vi "Bundle SV.vi"(8 "error in (no error)":errorcluster, 10 "Process Name":string="Flow Module 1", 11 "State Cluster in":T1={"Settings"={"Hardware Configuration"={"Tasks Array"=[]}, "Logging Configuration"={"Log File Base Path"=path ""}, "Feed Module Configuration"={"Cycle Period"=0.0, "Ismatech"={"VISA resource name"="", "Simulated?"=FALSE, "Pump Number"=0.0, "Reverse?"=FALSE}, "Masterflex"={"VISA resource name"="", "Simulated?"=FALSE, "Pump Number"=1.0, "Reverse?"=FALSE}, "Mettler"={"VISA resource name"="", "Simulated?"=FALSE}, "Bronkhorst M13 Flow Meter"={"VISA resource name"="", "Simulated?"=FALSE, "Smoothing Steps"=1}, "PID 2 Parameters"={"Input Device"=enum."Flowmeter", "Output Device"=enum."Ismatec ISM 831C", "Setpoint"=0.0, "PID gains"={"proportional gain (Kc)"=1.0, "integral time (Ti, min)"=0.01, "derivative time (Td, min)"=0.0}}, "Manual Entry"=0.0, "Auto?"=TRUE, "VICI Settings"={"VISA resource name"="", "Simulated?"=FALSE, "Pump Number"=0.0, "Reverse?"=FALSE}, "output range"={"output high"=100.0, "output low"=0.0}}, "Load Count"=0.0, "TT Configuration In"={"physical channels"="cDAQ2Mod4/ai0", "name to assign"="", "units"=10143}, "PT Configuration"={"physical channels"="cDAQ2Mod8/ai15", "name to assign"="Pressure", "units"=10342}}, "Shared Variables"={"PID 1 Process Variable"="PID1-Mettler Toledo Scale 1", "PID 1 Output"="PID1-Mettler Toledo Scale 1", "PID 1 Setpoint"="PID1-Setpoint", "PID 1 Setpoint SV refnum"="ni.var.psp://localhost/Flow Module 1/PID1-Setpoint", "PID 1 Process Variable SV refnum"="ni.var.psp://localhost/Flow Module 1/PID1-Setpoint", "PID 1 Output SV refnum"="ni.var.psp://localhost/Flow Module 1/PID1-Setpoint"}} {"Settings"."PT Configuration"."units" items=["Amps"=10342, "From Custom Scale"=10065]; "Settings"."TT Configuration In"."units" items=["Deg C"=10143, "Deg F"=10144, "Kelvins"=10325, "Deg R"=10145, "From Custom Scale"=10065]; "Settings"."Feed Module Configuration"."output range"."output low" min=0.0 max=100.0 format="%.2f"; "Settings"."Feed Module Configuration"."output range"."output high" format="%.2f"; "Settings"."Feed Module Configuration"."VICI Settings"."Pump Number" min=1.0 max=20.0 step=1.0; "Settings"."Feed Module Configuration"."PID 2 Parameters"."PID gains"."derivative time (Td, min)" format="%.3f"; "Settings"."Feed Module Configuration"."PID 2 Parameters"."PID gains"."integral time (Ti, min)" format="%.3f"; "Settings"."Feed Module Configuration"."PID 2 Parameters"."PID gains"."proportional gain (Kc)" format="%.3f"; "Settings"."Feed Module Configuration"."Bronkhorst M13 Flow Meter"."Smoothing Steps" min=1 step=1; "Settings"."Feed Module Configuration"."Masterflex"."Pump Number" min=1.0 max=20.0 step=1.0; "Settings"."Feed Module Configuration"."Ismatech"."Pump Number" min=1.0 max=20.0 step=1.0}) -> (0 "error out":errorcluster, 3 "State Cluster out":T1={"Settings"={"Hardware Configuration"={"Tasks Array"=[]}, "Logging Configuration"={"Log File Base Path"=path ""}, "Feed Module Configuration"={"Cycle Period"=0.0, "Ismatech"={"VISA resource name"="", "Simulated?"=FALSE, "Pump Number"=0.0, "Reverse?"=FALSE}, "Masterflex"={"VISA resource name"="", "Simulated?"=FALSE, "Pump Number"=1.0, "Reverse?"=FALSE}, "Mettler"={"VISA resource name"="", "Simulated?"=FALSE}, "Bronkhorst M13 Flow Meter"={"VISA resource name"="", "Simulated?"=FALSE, "Smoothing Steps"=1}, "PID 2 Parameters"={"Input Device"=enum."Flowmeter", "Output Device"=enum."Ismatec ISM 831C", "Setpoint"=0.0, "PID gains"={"proportional gain (Kc)"=1.0, "integral time (Ti, min)"=0.01, "derivative time (Td, min)"=0.0}}, "Manual Entry"=0.0, "Auto?"=TRUE, "VICI Settings"={"VISA resource name"="", "Simulated?"=FALSE, "Pump Number"=0.0, "Reverse?"=FALSE}, "output range"={"output high"=100.0, "output low"=0.0}}, "Load Count"=0.0, "TT Configuration In"={"physical channels"="cDAQ2Mod4/ai0", "name to assign"="", "units"=10143}, "PT Configuration"={"physical channels"="cDAQ2Mod8/ai15", "name to assign"="Pressure", "units"=10342}}, "Shared Variables"={"PID 1 Process Variable"="PID1-Mettler Toledo Scale 1", "PID 1 Output"="PID1-Mettler Toledo Scale 1", "PID 1 Setpoint"="PID1-Setpoint", "PID 1 Setpoint SV refnum"="ni.var.psp://localhost/Flow Module 1/PID1-Setpoint", "PID 1 Process Variable SV refnum"="ni.var.psp://localhost/Flow Module 1/PID1-Setpoint", "PID 1 Output SV refnum"="ni.var.psp://localhost/Flow Module 1/PID1-Setpoint"}} {"Settings"."PT Configuration"."units" items=["Amps"=10342, "From Custom Scale"=10065]; "Settings"."TT Configuration In"."units" items=["Deg C"=10143, "Deg F"=10144, "Kelvins"=10325, "Deg R"=10145, "From Custom Scale"=10065]; "Settings"."Feed Module Configuration"."output range"."output low" min=0.0 max=100.0 format="%.2f"; "Settings"."Feed Module Configuration"."output range"."output high" format="%.2f"; "Settings"."Feed Module Configuration"."VICI Settings"."Pump Number" min=1.0 max=20.0 step=1.0; "Settings"."Feed Module Configuration"."PID 2 Parameters"."PID gains"."derivative time (Td, min)" format="%.3f"; "Settings"."Feed Module Configuration"."PID 2 Parameters"."PID gains"."integral time (Ti, min)" format="%.3f"; "Settings"."Feed Module Configuration"."PID 2 Parameters"."PID gains"."proportional gain (Kc)" format="%.3f"; "Settings"."Feed Module Configuration"."Bronkhorst M13 Flow Meter"."Smoothing Steps" min=1 step=1; "Settings"."Feed Module Configuration"."Masterflex"."Pump Number" min=1.0 max=20.0 step=1.0; "Settings"."Feed Module Configuration"."Ismatech"."Pump Number" min=1.0 max=20.0 step=1.0})   [LabVIEW 2021, in "Scale Module.lvlib"]
uses:
  Scale Module.lvlib
  Shared Variables/Dynamic Shared Variables.lvlib
  Controls/Scale Module Shared Variable Cluster.ctl
  Acquisition/Hardware Configuration.ctl
  DAQ/DAQ.lvlib
  Logging/Logging Configuration.ctl
  Logging/Logging.lvlib
  Controls/Scale Module Settings Cluster.ctl
  Settings/Settings.ctl
  Settings/Settings.lvlib
  Controls/Scale Module State Cluster.ctl
  Masterflex 7550-30/Controls/Settings Cluster.ctl
  Masterflex 7550-30/Masterflex 7550-30.lvlib
  Mettler Toledo/Controls/Settings Cluster.ctl
  Mettler Toledo/Mettler Toledo.lvlib
  Bronkhorst M13 Flow Meter/Settings Cluster.ctl
  Bronkhorst M13 Flow Meter/Bronkhorst M13 Flow Meter.lvlib
  Measure Instrument/PID Input Enum.ctl
  Measure Instrument/PID 2 Output Enum.ctl
  Measure Instrument/PID 2 Parameters Cluster.ctl
  Ismatec ISM 831C/Controls/Ismatech Settings Cluster.ctl
  Pressure Sensor/PT Configuration.ctl
  Pressure Sensor/Pressure.lvlib
  Acquisition/Task Cluster.ctl
  VICI M50/VICI Settings.ctl
panel:
  # "Output Instruments"
  # "Input Instruments"
  # "Output Instruments"
  # "Input Instruments"
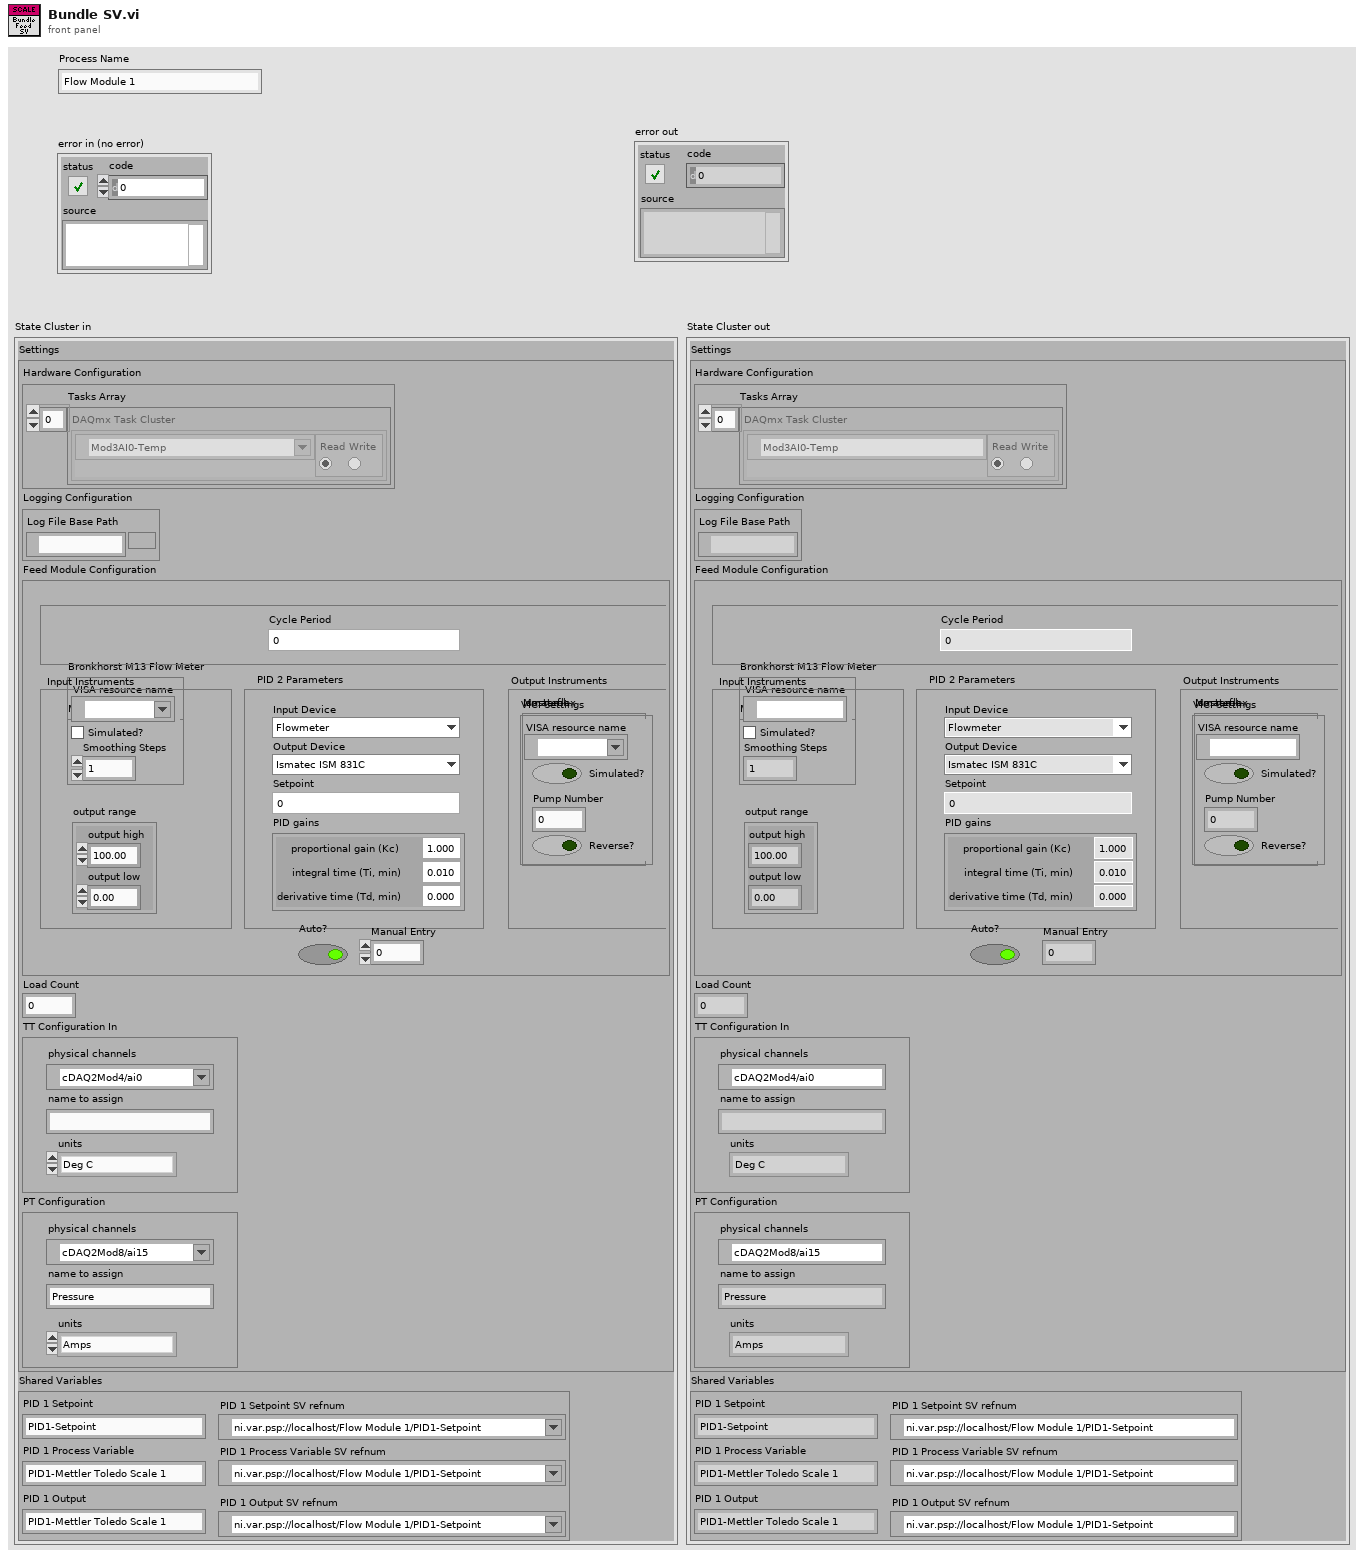
[diagram p1: front panel]
types:
  T1 = typedef "Scale Module.lvlib/Scale Module State Cluster.ctl" = cluster{"Settings":T2, "Shared Variables":T16}
  T2 = typedef "Settings.lvlib/Settings.ctl" = cluster{"Hardware Configuration":T3, "Logging Configuration":T5, "Feed Module Configuration":T6, "Load Count":dbl, "TT Configuration In":cluster{"physical channels":tag, "name to assign":string, "units":i32}, "PT Configuration":T15}
  T3 = typedef "DAQ.lvlib/Hardware Configuration.ctl" = cluster{"Tasks Array":T4[]}
  T4 = typedef "Task Cluster.ctl" = cluster{"DAQmx Task":refnum<k21>, "Read-Write Radio":enum32{"Read", "Write"}}
  T5 = typedef "Logging.lvlib/Logging Configuration.ctl" = cluster{"Log File Base Path":path}
  T6 = typedef "Scale Module.lvlib/Scale Module Settings Cluster.ctl" = cluster{"Cycle Period":dbl, "Ismatech":T7, "Masterflex":T8, "Mettler":T9, "Bronkhorst M13 Flow Meter":T10, "PID 2 Parameters":T11, "Manual Entry":dbl, "Auto?":bool, "VICI Settings":T14, "output range":cluster{"output high":dbl, "output low":dbl}}
  T7 = typedef "Ismatec ISM 831C.lvlib/Ismatech Settings Cluster.ctl" = cluster{"VISA resource name":refnum<visa-resource-name>, "Simulated?":bool, "Pump Number":dbl, "Reverse?":bool}
  T8 = typedef "Masterflex 7550-30.lvlib/Settings Cluster.ctl" = cluster{"VISA resource name":refnum<visa-resource-name>, "Simulated?":bool, "Pump Number":dbl, "Reverse?":bool}
  T9 = typedef "Mettler Toledo.lvlib/Settings Cluster.ctl" = cluster{"VISA resource name":refnum<visa-resource-name>, "Simulated?":bool}
  T10 = typedef "Bronkhorst M13 Flow Meter.lvlib/Settings Cluster.ctl" = cluster{"VISA resource name":refnum<visa-resource-name>, "Simulated?":bool, "Smoothing Steps":i32}
  T11 = typedef "PID 2 Parameters Cluster.ctl" = cluster{"Input Device":T12, "Output Device":T13, "Setpoint":dbl, "PID gains":cluster{"proportional gain (Kc)":dbl, "integral time (Ti, min)":dbl, "derivative time (Td, min)":dbl}}
  T12 = typedef "PID Input Enum.ctl" = enum16{"Default", "Flowmeter", "Scale Rate of Change"}
  T13 = typedef "PID 2 Output Enum.ctl" = enum16{"Default", "Ismatec ISM 4308", "Ismatec ISM 831C", "Masterflex 7550-30", "VICI M6", "VICI M50", "Tacmina QI", "KNF SIMDOS", "ASIA Type C", "FLOM UI-22-11", "SSI PR/LD", "SSI P40", "Masterflex 75211-70"}
  T14 = typedef "VICI Settings.ctl" = cluster{"VISA resource name":refnum<visa-resource-name>, "Simulated?":bool, "Pump Number":dbl, "Reverse?":bool}
  T15 = typedef "Pressure.lvlib/PT Configuration.ctl" = cluster{"physical channels":tag, "name to assign":string, "units":i32}
  T16 = typedef "Scale Module.lvlib/Scale Module Shared Variable Cluster.ctl" = cluster{"PID 1 Process Variable":string, "PID 1 Output":string, "PID 1 Setpoint":string, "PID 1 Setpoint SV refnum":refnum<k21>, "PID 1 Process Variable SV refnum":refnum<k21>, "PID 1 Output SV refnum":refnum<k21>}
  T17 = cluster{"enable? (F)":bool, "name":string, "alarm type":enum16{"HI_HI", "HI", "LO", "LO_LO"}, "level/change":dbl, "deadband/time":dbl, "priority":u32, "ack type":enum16{"Auto", "User", "None", "Each Occurrence"}, "area":string, "description":string, "log? (T)":bool}
  T18 = typedef "Hardware.lvclass/Configuration Cluster.ctl" = cluster{"VISA resource name":refnum<visa-resource-name>, "Measure Period (ms)":i32, "Instrument":T19, "Ismatech Settings":T20, "Masterflex Settings":T21, "Mettler Settings":T22, "Bronkhorst M13 Flow Meter Settings":T23, "PID 2 Parameters":T24}
  T19 = typedef "Feed Module.lvlib/Measure Instrument Enum.ctl" = enum16{"None", "Mettler Toledo Scale", "Bronkhorst M13 Flow Meter"}
  T20 = typedef "Ismatec ISM 831C.lvlib/Imatech Settings Cluster.ctl" = cluster{"VISA resource name":refnum<visa-resource-name>}
  T21 = typedef "Masterflex 7550-30.lvlib/Settings Cluster.ctl" = cluster{"VISA resource name":refnum<visa-resource-name>}
  T22 = typedef "Mettler Toledo.lvlib/Settings Cluster.ctl" = cluster{"VISA resource name":refnum<visa-resource-name>}
  T23 = typedef "Bronkhorst M13 Flow Meter.lvlib/Settings Cluster.ctl" = cluster{"VISA resource name":refnum<visa-resource-name>}
  T24 = typedef "PID 2 Parameters Cluster.ctl" = cluster{"Input Device":T25, "Output Device":T26, "Setpoint":dbl, "PID gains":cluster{"proportional gain (Kc)":dbl, "integral time (Ti, min)":dbl, "derivative time (Td, min)":dbl}}
  T25 = typedef "PID Input Enum.ctl" = enum16{"Flowmeter", "Scale Rate of Change"}
  T26 = typedef "PID 2 Output Enum.ctl" = enum16{"Ismatec ISM 831C", "Masterflex 7550-30"}
  T27 = cluster{"enable? (F)":bool, "name":string, "alarm type":enum16{"HI_HI", "HI", "LO", "LO_LO"}, "level/change":dbl, "deadband/time":dbl, "priority":u32, "ack type":enum16{"Auto", "User", "None", "Each Occurrence"}, "area":string, "description":string, "log? (T)":bool}[]
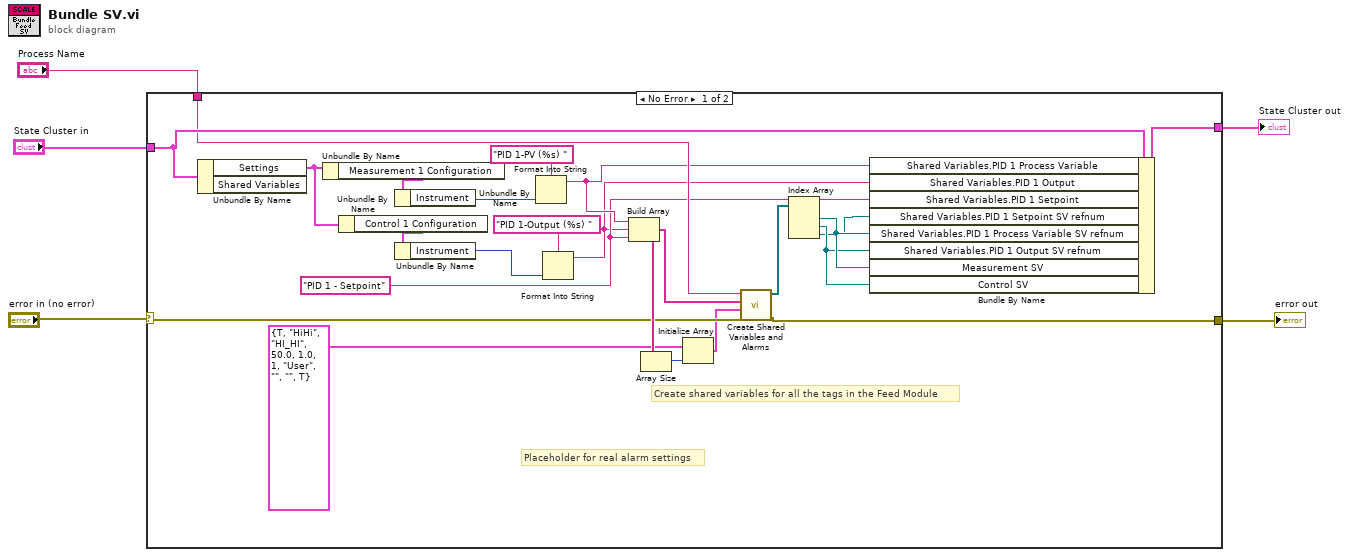
[diagram p0: block diagram]
diagram:
  n1 = case shown="No Error" "error in (no error)" {
    selector: "error in (no error)" -> [w23 w30]
    tunnel: "Process Name" -> [w27 _]
    tunnel: [w22 w30] -> w3
    tunnel: "State Cluster in" -> [w28 w29]
    tunnel: [w20 w29] -> w1
    frame No Error {
      w10 = "PID 1 - Setpoint" ("element")
      # "Create shared variables for all the tags in the Feed Module"
      # "Placeholder for real alarm settings"
      n2 = Unbundle By Name(w28) -> ("Settings"=w13:T2)  [unwired: 1 out]
      n3 = Unbundle By Name(w13) -> ("Measurement 1 Configuration"=w18:T18)
      n4 = Unbundle By Name(w13) -> ("Control 1 Configuration"=w14:T18)
      n5 = Unbundle By Name(w18) -> ("Instrument"=w16:T19)
      n6 = Unbundle By Name(w14) -> ("Instrument"=w11:T19)
      n7 = Format Into String(format string="PID 1-PV (%s) ", w16) -> (resulting string=w15:string)  [unwired: 2 in, 1 out]
      n8 = Format Into String(format string="PID 1-Output (%s) ", w11) -> (resulting string=w9:string)  [unwired: 2 in, 1 out]
      n9 = Build Array(w15, w9, w10) -> (w26:string[])
      n10 = Array Size(array=w26) -> (size(s)=w25:i32)
      n11 = Initialize Array(T17 {"enable? (F)"=TRUE, "name"="HiHi", "alarm type"=enum."HI_HI", "level/change"=50.0, "deadband/time"=1.0, "priority"=1, "ack type"=enum."User", "area"="", "description"="", "log? (T)"=TRUE} ("numeric alarm settings"), w25) -> (w19:T27)
      n12 = call "Create Shared Variables and Alarms.vi"("error in (no error)"=w23, "Alarm Settings"=w19, "Shared Variable Names"=w26, "Process Name"=w27) -> ("error out"=w22:errorcluster, "Shared Variable refnums"=w21:refnum<k21>[])  [unwired: 6 in]
      n13 = Index Array(array=w21) -> (element #1=w8:refnum<k21>, element #2=w7:refnum<k21>, element #3=w6:refnum<k21>)  [unwired: 3 in]
      n14 = Bundle By Name(cluster=w28, "Shared Variables.PID 1 Process Variable"=w15, "Shared Variables.PID 1 Output"=w9, "Shared Variables.PID 1 Setpoint"=w10, "Shared Variables.PID 1 Setpoint SV refnum"=w6, "Shared Variables.PID 1 Process Variable SV refnum"=w8, "Shared Variables.PID 1 Output SV refnum"=w7, "Measurement SV"=w8, "Control SV"=w7) -> (w20:T1)
    }
    frame Error {
    }
  }
  "error out" <- w3
  "State Cluster out" <- w1
